vi "SetTOREG_SD.vi"(0 "fkt":u8) -> ()   [LabVIEW 2015]
uses:
  DLL/ESLSCDLL.dll
panel:
  # "if (fkt==0)set to REG -> XCK\nif (fkt==1)set to REG -> OutTrig\nif (fkt==2)set to FFRead\nif (fkt==3)set to IRArea read (VON)\nif (fkt==4)set to EC\nif (fkt==5)set to DAT"
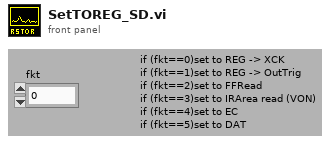
[diagram p1: front panel]
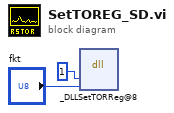
[diagram p0: block diagram]
diagram:
  n1 = dll-call lib="G:/SD/TRANCON-2015/DLL/ESLSCDLL.dll" fn="_DLLSetTORReg@8" ("lwlscdll.dll:DLLRsTOREG")("drv"=u32 1, "fkt"="fkt") -> ()  [unwired: 6 in, 2 out]
